vi "Settings Dialog.vi"(8 "error in (no error)":errorcluster, 11 "Settings in":T1={"Hardware Configuration"={"DAQmx Channel"="", "Max Input"=10.0, "Min Input"=-10.0, "Sample Rate"=1000.0, "DAQmx Task"="", "Fichier de simulation"=path "", "Source"=enum."Simulation"}, "Logging Configuration"={"Log File Base Path"=path "", "DAQ Log TDMS File Reference"=refnum, "Samples to Save"=0, "Trigger - Time"=0, "Trigger - Threshold"=0.0, "Trigger - Channel"=0, "Enable Time Trigger"=FALSE, "Enable Threshold Trigger"=FALSE, "Always Log"=FALSE, "Session Name"="", "Estimate Batch Size"=0, "Estimate Filepath"=path ""}}) -> (0 "error out":errorcluster, 1 "Cancelled?":bool=TRUE, 2 "UI Refresh Needed?":bool, 3 "Settings out":T1={"Hardware Configuration"={"DAQmx Channel"="", "Max Input"=10.0, "Min Input"=-10.0, "Sample Rate"=1000.0, "DAQmx Task"="", "Fichier de simulation"=path "", "Source"=enum."Simulation"}, "Logging Configuration"={"Log File Base Path"=path "C:/Users/jpassiak/Documents/LabVIEW Data/Logged Data.tdms", "DAQ Log TDMS File Reference"=refnum, "Samples to Save"=0, "Trigger - Time"=0, "Trigger - Threshold"=0.0, "Trigger - Channel"=0, "Enable Time Trigger"=FALSE, "Enable Threshold Trigger"=FALSE, "Always Log"=FALSE, "Session Name"="", "Estimate Batch Size"=0, "Estimate Filepath"=path ""}})   [LabVIEW 2019, in "Settings.lvlib"]
doc: "Dialog for selecting user specified settings."
uses:
  Settings.lvlib
  Settings.ctl
  Acquisition/Hardware Configuration.ctl
  Logging/Logging Configuration.ctl
  <vilib>/Utility/xml.llb/Write to XML File(string).vi
  Acquisition/Acquisition.lvlib
  Logging/Logging.lvlib
panel:
  in  "Source":enum16{"Simulation", "DAQ"}(ring)
  in  "Fichier de simulation":path
  in  "Nom de la session":string
  in  "Nombre d'estimé enregistré\npar transaction":i32
  in  "Log when triggered":bool
  in  "Trigger Channel":u32
  in  "Taille d'enregistrement":u32=500 min=1
  in  "Trigger Threshold (V)":dbl=2.0
  in  "Trigger Time (min)":u32=1
  in  "Enable Threshold Trigger (V):":bool
  in  "Enable Time Trigger (min):":bool
  in  "Always Log":bool
  in  "Fréquence d'échantillonage":dbl=1000.0
  in  "Minimum DAQ virtuel":dbl=-10.0
  in  "Maximum DAQ virtuel":dbl=10.0
  in  "Dossier temporaire":path
  in  "Cancel Button":bool
  in  "OK Button":bool
  # "Acquisition"
  # "Non visible portion of dialog (needed for connector pane)."
  # "Trigger"
  # "Journalisation"
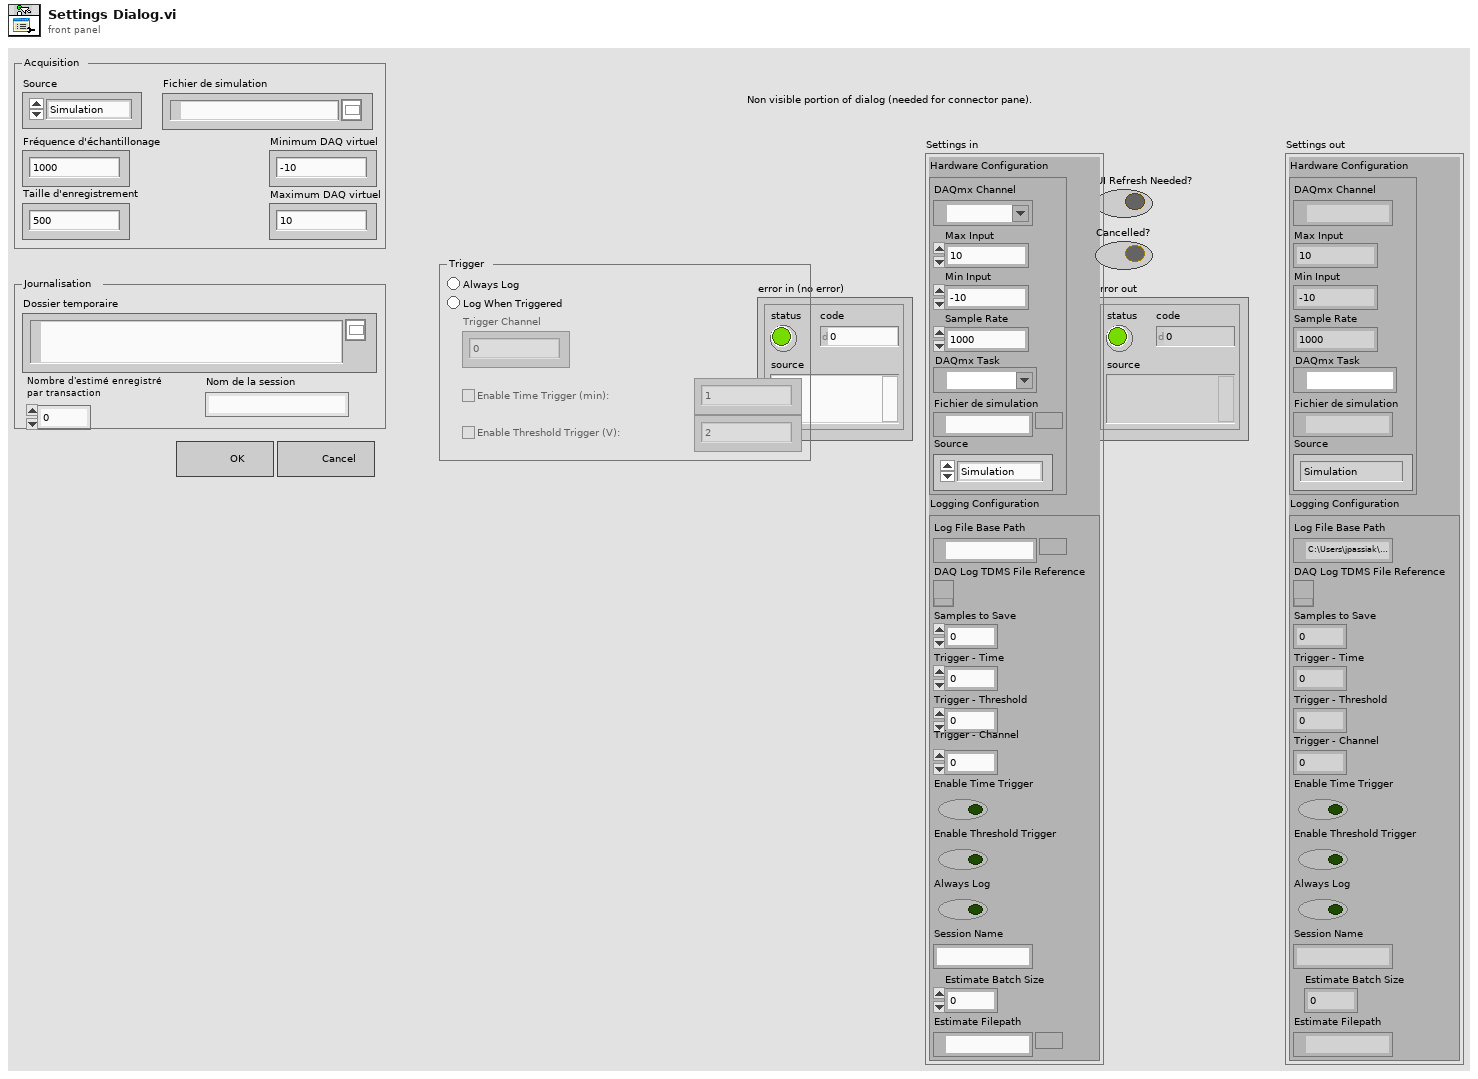
[diagram p1: front panel]
types:
  T1 = typedef "Settings.lvlib/Settings.ctl" = cluster{"Hardware Configuration":T2, "Logging Configuration":T3}
  T2 = typedef "Acquisition.lvlib/Hardware Configuration.ctl" = cluster{"DAQmx Channel":tag, "Max Input":dbl, "Min Input":dbl, "Sample Rate":dbl, "DAQmx Task":refnum<k21>, "Fichier de simulation":path, "Source":enum16{"Simulation", "DAQ"}}
  T3 = typedef "Logging.lvlib/Logging Configuration.ctl" = cluster{"Log File Base Path":path, "DAQ Log TDMS File Reference":refnum<k34>, "Samples to Save":u32, "Trigger - Time":u32, "Trigger - Threshold":dbl, "Trigger - Channel":u32, "Enable Time Trigger":bool, "Enable Threshold Trigger":bool, "Always Log":bool, "Session Name":string, "Estimate Batch Size":i32, "Estimate Filepath":path}
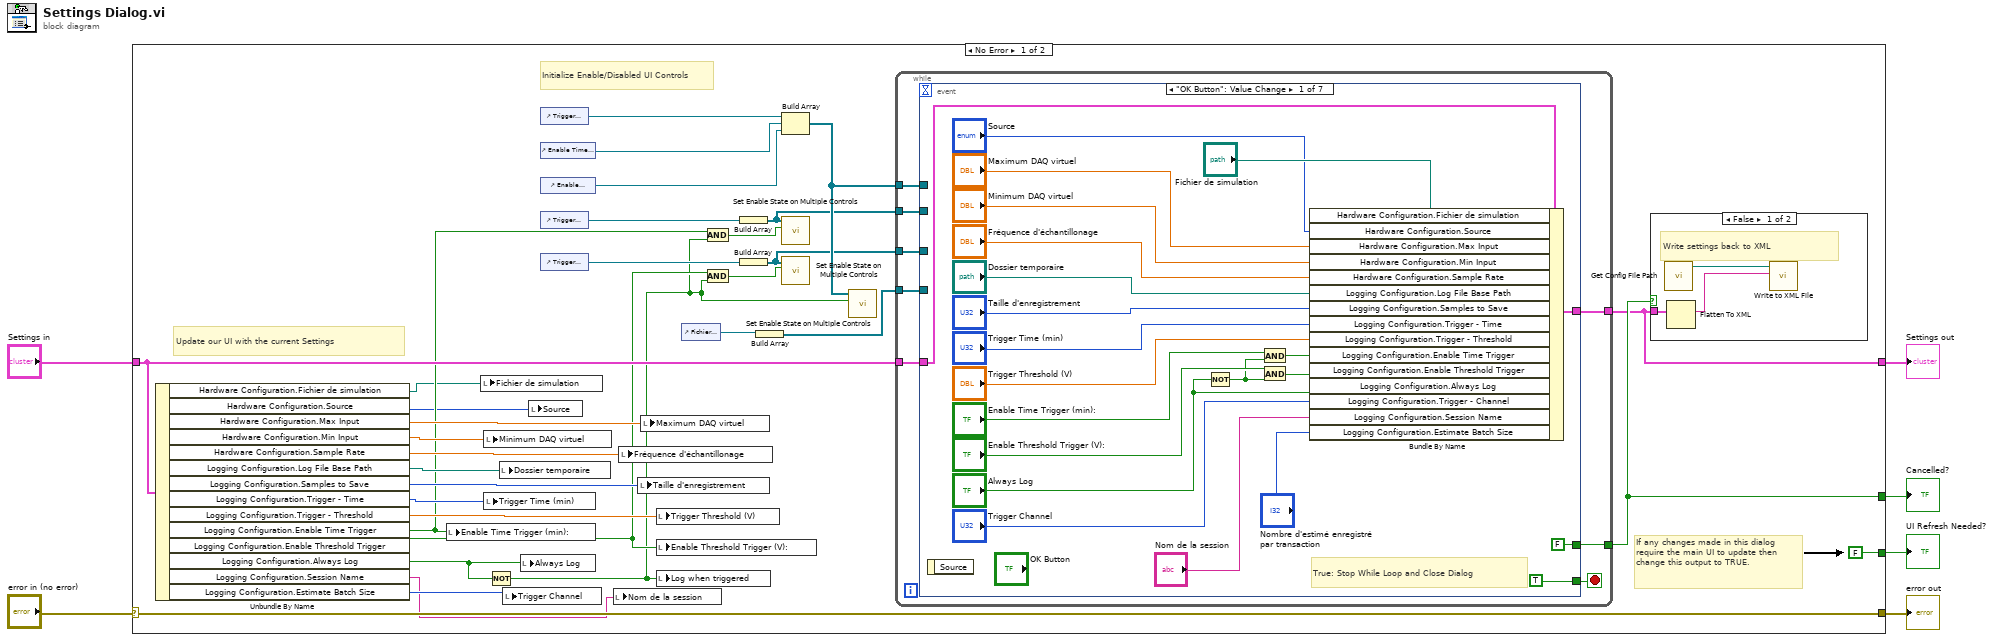
[diagram p0: block diagram]
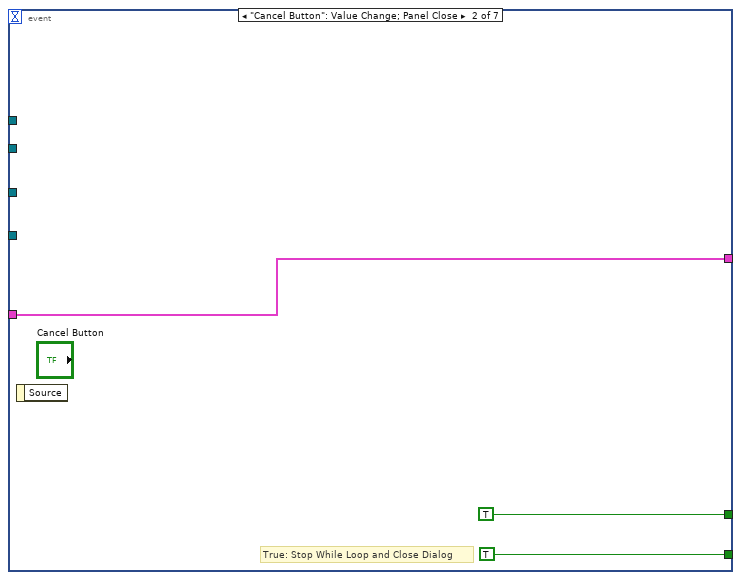
[diagram p2: hidden frame]
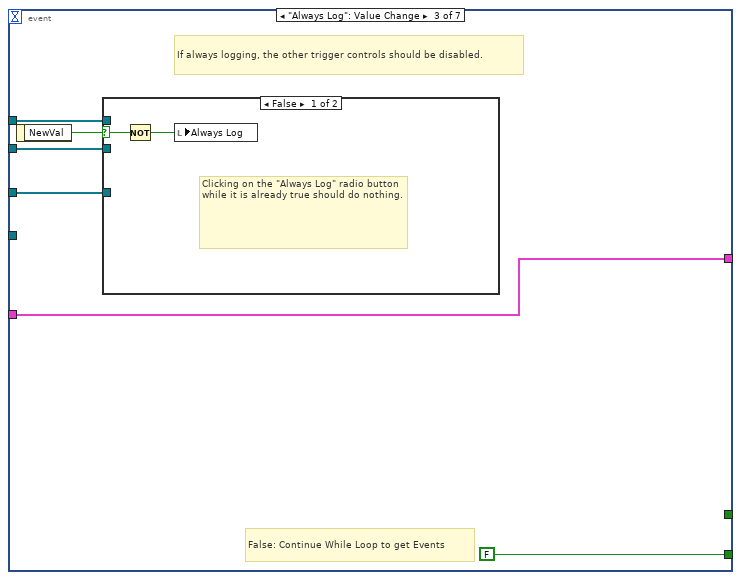
[diagram p3: hidden frame]
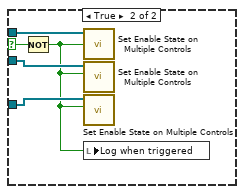
[diagram p4: hidden frame]
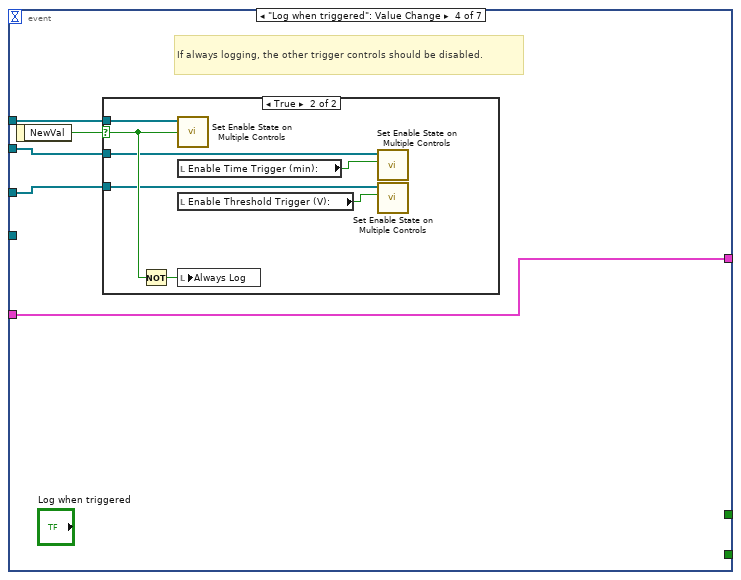
[diagram p5: hidden frame]
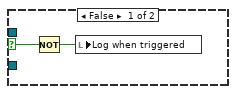
[diagram p6: hidden frame]
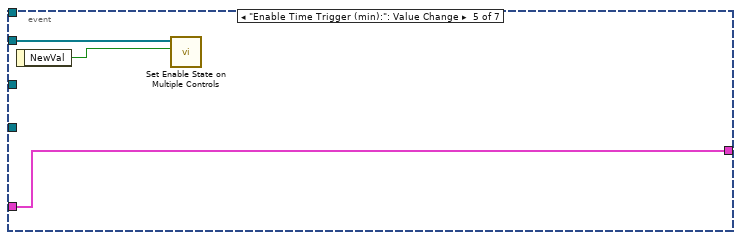
[diagram p7: hidden frame]
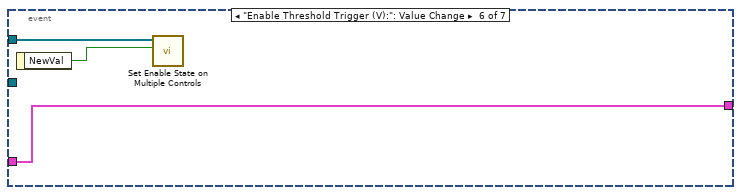
[diagram p8: hidden frame]
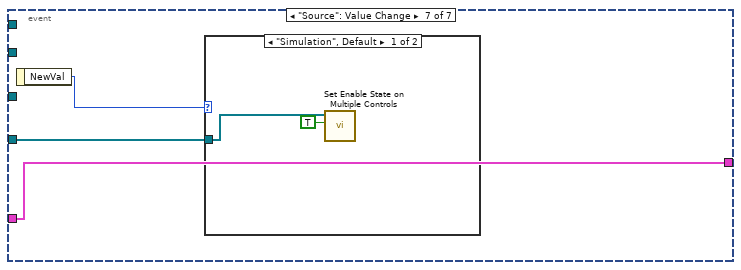
[diagram p9: hidden frame]
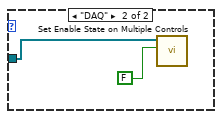
[diagram p10: hidden frame]
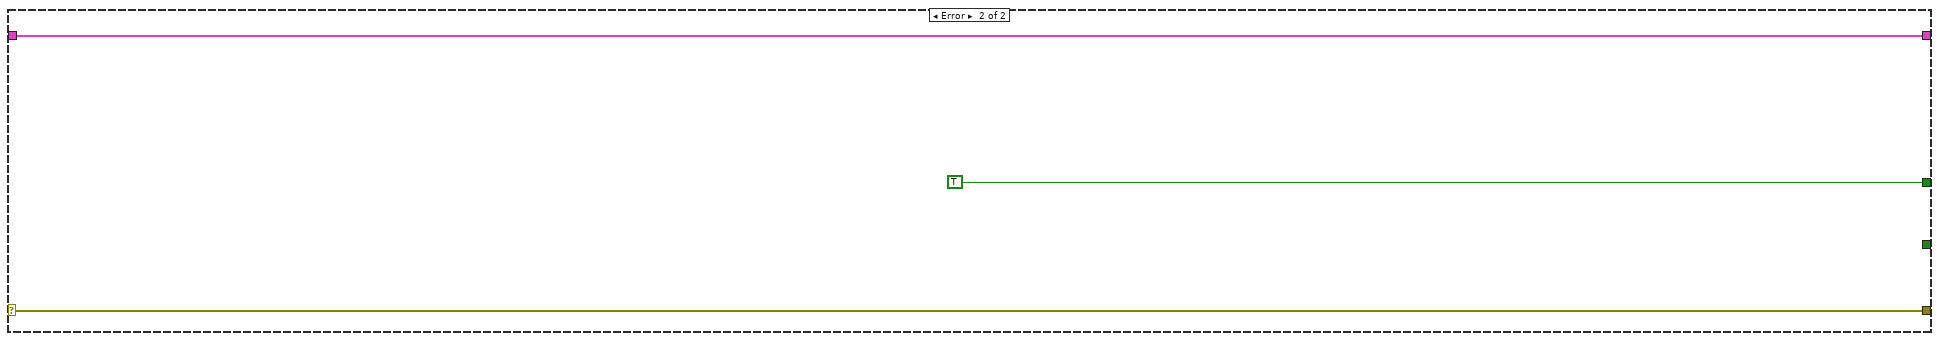
[diagram p12: hidden frame]
diagram:
  n1 = case shown="No Error" "error in (no error)" {
    selector: "error in (no error)" -> [w38 w117]
    tunnel: [w38 w117] -> w6
    tunnel: "Settings in" -> [w25 w116]
    tunnel: [w35 w116] -> w4
    tunnel: [FALSE ("UI Refresh Needed?") _] -> w3
    tunnel: [w36 TRUE ("UI Refresh Needed?")] -> w2
    frame No Error {
      # "Update our UI with the current Settings"
      # "Initialize Enable/Disabled UI Controls"
      # "If any changes made in this dialog require the main UI to update then change this output to TRUE."
      n2 = Unbundle By Name(w25) -> ("Hardware Configuration.Fichier de simulation"=w10:path, "Hardware Configuration.Source"=w9:enum16{"Simulation", "DAQ"}, "Hardware Configuration.Max Input"=w32:dbl, "Hardware Configuration.Min Input"=w33:dbl, "Hardware Configuration.Sample Rate"=w34:dbl, "Logging Configuration.Log File Base Path"=w31:path, "Logging Configuration.Samples to Save"=w30:u32, "Logging Configuration.Trigger - Time"=w29:u32, "Logging Configuration.Trigger - Threshold"=w28:dbl, "Logging Configuration.Enable Time Trigger"=w17:bool, "Logging Configuration.Enable Threshold Trigger"=w16:bool, "Logging Configuration.Always Log"=w27:bool, "Logging Configuration.Session Name"=w11:string, "Logging Configuration.Estimate Batch Size"=w12:i32)
      n3 = local write "Enable Time Trigger (min):"(w17) -> ()
      n4 = local write "Fichier de simulation"(w10) -> ()
      n5 = local write "Minimum DAQ virtuel"(w33) -> ()
      n6 = local write "Trigger Time (min)"(w29) -> ()
      n7 = Not(x=w27) -> (.not. x?=w13:bool)
      n8 = local write "Dossier temporaire"(w31) -> ()
      n9 = local write "Trigger Channel"(w12) -> ()
      n10 = local write "Always Log"(w27) -> ()
      n11 = local write "Source"(w9) -> ()
      n12 = control-ref of="Trigger Channel"() -> (w24:refnum<vi>)
      n13 = control-ref of="Enable Time Trigger (min):"() -> (w23:refnum<vi>)
      n14 = control-ref of="Enable Threshold Trigger (V):"() -> (w22:refnum<vi>)
      n15 = control-ref of="Trigger Time (min)"() -> (w21:refnum<vi>)
      n16 = control-ref of="Trigger Threshold (V)"() -> (w20:refnum<vi>)
      n17 = local write "Nom de la session"(w11) -> ()
      n18 = local write "Fréquence d'échantillonage"(w34) -> ()
      n19 = local write "Taille d'enregistrement"(w30) -> ()
      n20 = local write "Maximum DAQ virtuel"(w32) -> ()
      n21 = local write "Trigger Threshold (V)"(w28) -> ()
      n22 = local write "Enable Threshold Trigger (V):"(w16) -> ()
      n23 = local write "Log when triggered"(w13) -> ()
      n24 = control-ref of="Fichier de simulation"() -> (w8:refnum<vi>)
      n25 = And(x=w17, y=w13) -> (x .and. y?=w19:bool)
      n26 = And(x=w16, y=w13) -> (x .and. y?=w18:bool)
      n27 = Build Array(w21) -> (w15:refnum<vi>[])
      n28 = Build Array(w20) -> (w14:refnum<vi>[])
      n29 = Build Array(w8) -> (w7:refnum<vi>[])
      n30 = Build Array(w24, w23, w22) -> (w26:refnum<vi>[])
      n31 = call "Set Enable State on Multiple Controls.vi"("Enable?"=w19, "Controls"=w15) -> ()  [unwired: 10 in]
      n32 = call "Set Enable State on Multiple Controls.vi"("Enable?"=w18, "Controls"=w14) -> ()  [unwired: 10 in]
      n33 = call "Set Enable State on Multiple Controls.vi"("Enable?"=w13, "Controls"=w26) -> ()  [unwired: 10 in]
      n34 = while {
        tunnel: [w46] -> w36
        tunnel: [w45] -> w35
        tunnel: w25 -> [w44]
        tunnel: w26 -> [w42]
        tunnel: w15 -> [w41]
        tunnel: w14 -> [w40]
        tunnel: w7 -> [w39]
        stop <- w43 stop-if-true
        n35 = event shown="[0] \"OK Button\": Value Change" {
          selector: _ -> [_ _ _ _ _ _ _]
          dyn-events: _ -> [_ _ _ _ _ _ _]
          timeout: _ -> [_ _ _ _ _ _ _]
          tunnel: [w66 w71 w77 w89 w101 w104 w107] -> w45
          tunnel: w44 -> [w65 w71 w77 w89 w101 w104 w107]
          tunnel: [FALSE ("UI Refresh Needed?") TRUE ("UI Refresh Needed?") _ _ _ _ _] -> w46
          tunnel: [TRUE TRUE FALSE _ _ _ _] -> w43
          tunnel: w42 -> [_ _ w75 w88 _ _ _]
          tunnel: w41 -> [_ _ w73 w86 w100 _ _]
          tunnel: w40 -> [_ _ w72 w85 _ w103 _]
          tunnel: w39 -> [_ _ _ _ _ _ w105]
          event "OK Button": Value Change {
            # "True: Stop While Loop and Close Dialog"
            n36 = event-data() -> ()  [unwired: 1 in, 1 out]
            n37 = Not(x="Always Log") -> (.not. x?=w51:bool)
            n38 = And(x="Enable Time Trigger (min):", y=w51) -> (x .and. y?=w52:bool)
            n39 = And(x="Enable Threshold Trigger (V):", y=w51) -> (x .and. y?=w54:bool)
            n40 = Bundle By Name(cluster=w65, "Hardware Configuration.Fichier de simulation"="Fichier de simulation", "Hardware Configuration.Source"="Source", "Hardware Configuration.Max Input"="Maximum DAQ virtuel", "Hardware Configuration.Min Input"="Minimum DAQ virtuel", "Hardware Configuration.Sample Rate"="Fréquence d'échantillonage", "Logging Configuration.Log File Base Path"="Dossier temporaire", "Logging Configuration.Samples to Save"="Taille d'enregistrement", "Logging Configuration.Trigger - Time"="Trigger Time (min)", "Logging Configuration.Trigger - Threshold"="Trigger Threshold (V)", "Logging Configuration.Enable Time Trigger"=w52, "Logging Configuration.Enable Threshold Trigger"=w54, "Logging Configuration.Always Log"="Always Log", "Logging Configuration.Trigger - Channel"="Trigger Channel", "Logging Configuration.Session Name"="Nom de la session", "Logging Configuration.Estimate Batch Size"="Nombre d'estimé enregistré\npar transaction") -> (w66:T1)
          }
          event "Cancel Button": Value Change; Panel Close {
            # "True: Stop While Loop and Close Dialog"
            n41 = event-data() -> ()  [unwired: 1 in, 1 out]
          }
          event "Always Log": Value Change {
            # "False: Continue While Loop to get Events"
            # "If always logging, the other trigger controls should be disabled."
            n42 = event-data() -> ("NewVal"=w74:bool)  [unwired: 1 in]
            n43 = case shown="False" w74 {
              selector: w74 -> [w79 w84]
              tunnel: w75 -> [_ w83]
              tunnel: w73 -> [_ w82]
              tunnel: w72 -> [_ w81]
              frame False {
                # "Clicking on the \"Always Log\" radio button while it is already true should do nothing."
                n44 = Not(x=w79) -> (.not. x?=w78:bool)
                n45 = local write "Always Log"(w78) -> ()
              }
              frame True {
                n46 = Not(x=w84) -> (.not. x?=w80:bool)
                n47 = call "Set Enable State on Multiple Controls.vi"("Enable?"=w80, "Controls"=w83) -> ()  [unwired: 10 in]
                n48 = call "Set Enable State on Multiple Controls.vi"("Enable?"=w80, "Controls"=w82) -> ()  [unwired: 10 in]
                n49 = call "Set Enable State on Multiple Controls.vi"("Enable?"=w80, "Controls"=w81) -> ()  [unwired: 10 in]
                n50 = local write "Log when triggered"(w80) -> ()
              }
            }
          }
          event "Log when triggered": Value Change {
            # "If always logging, the other trigger controls should be disabled."
            n51 = event-data() -> ("NewVal"=w87:bool)  [unwired: 1 in]
            n52 = case shown="True" w87 {
              selector: w87 -> [w91 w97]
              tunnel: w88 -> [_ w98]
              tunnel: w86 -> [_ w95]
              tunnel: w85 -> [_ w94]
              frame False {
                n53 = Not(x=w91) -> (.not. x?=w90:bool)
                n54 = local write "Log when triggered"(w90) -> ()
              }
              frame True {
                n55 = Not(x=w97) -> (.not. x?=w96:bool)
                n56 = call "Set Enable State on Multiple Controls.vi"("Enable?"=w97, "Controls"=w98) -> ()  [unwired: 10 in]
                n57 = local read "Enable Time Trigger (min):"() -> (w92:bool)
                n58 = local read "Enable Threshold Trigger (V):"() -> (w93:bool)
                n59 = local write "Always Log"(w96) -> ()
                n60 = call "Set Enable State on Multiple Controls.vi"("Enable?"=w92, "Controls"=w95) -> ()  [unwired: 10 in]
                n61 = call "Set Enable State on Multiple Controls.vi"("Enable?"=w93, "Controls"=w94) -> ()  [unwired: 10 in]
              }
            }
          }
          event "Enable Time Trigger (min):": Value Change {
            n62 = event-data() -> ("NewVal"=w99:bool)  [unwired: 1 in]
            n63 = call "Set Enable State on Multiple Controls.vi"("Enable?"=w99, "Controls"=w100) -> ()  [unwired: 10 in]
          }
          event "Enable Threshold Trigger (V):": Value Change {
            n64 = event-data() -> ("NewVal"=w102:bool)  [unwired: 1 in]
            n65 = call "Set Enable State on Multiple Controls.vi"("Enable?"=w102, "Controls"=w103) -> ()  [unwired: 10 in]
          }
          event "Source": Value Change {
            n66 = event-data() -> ("NewVal"=w106:enum16{"Simulation", "DAQ"})  [unwired: 1 in]
            n67 = case shown="\"Simulation\", Default" w106 {
              tunnel: w105 -> [w109 w111]
              frame "Simulation", Default {
                n68 = call "Set Enable State on Multiple Controls.vi"("Enable?"=TRUE, "Controls"=w109) -> ()  [unwired: 10 in]
              }
              frame "DAQ" {
                n69 = call "Set Enable State on Multiple Controls.vi"("Enable?"=FALSE, "Controls"=w111) -> ()  [unwired: 10 in]
              }
            }
          }
        }
      }
      n70 = case shown="False" w36 {
        tunnel: w35 -> [w113 _]
        frame False {
          # "Write settings back to XML"
          n71 = call "Get Config File Path.vi"() -> ("XML File Path"=w114:path)  [unwired: 10 in, 1 out]
          n72 = Flatten To XML(anything=w113) -> (xml string=w112:string)
          n73 = call-poly <vilib>:"Write to XML File.vi"("XML Input"=w112, "XML File Path"=w114) -> ()  [unwired: 7 in, 3 out]
        }
        frame True {
        }
      }
    }
    frame Error {
    }
  }
  "UI Refresh Needed?" <- w3
  "error out" <- w6
  "Settings out" <- w4
  "Cancelled?" <- w2
